vi "Menu-status.vi"(6 "File and Help Menu":bool, 7 "Menu Refnum":refnum<k9>, 8 "Temperature Controller Initialized":bool, 9 "Stage Initialized":bool, 10 "Monochromator Initialized":bool, 11 "CCD Initialized":bool) -> ()   [LabVIEW 2009]
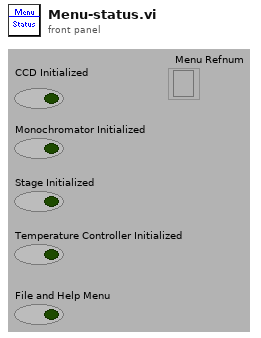
[diagram p1: front panel]
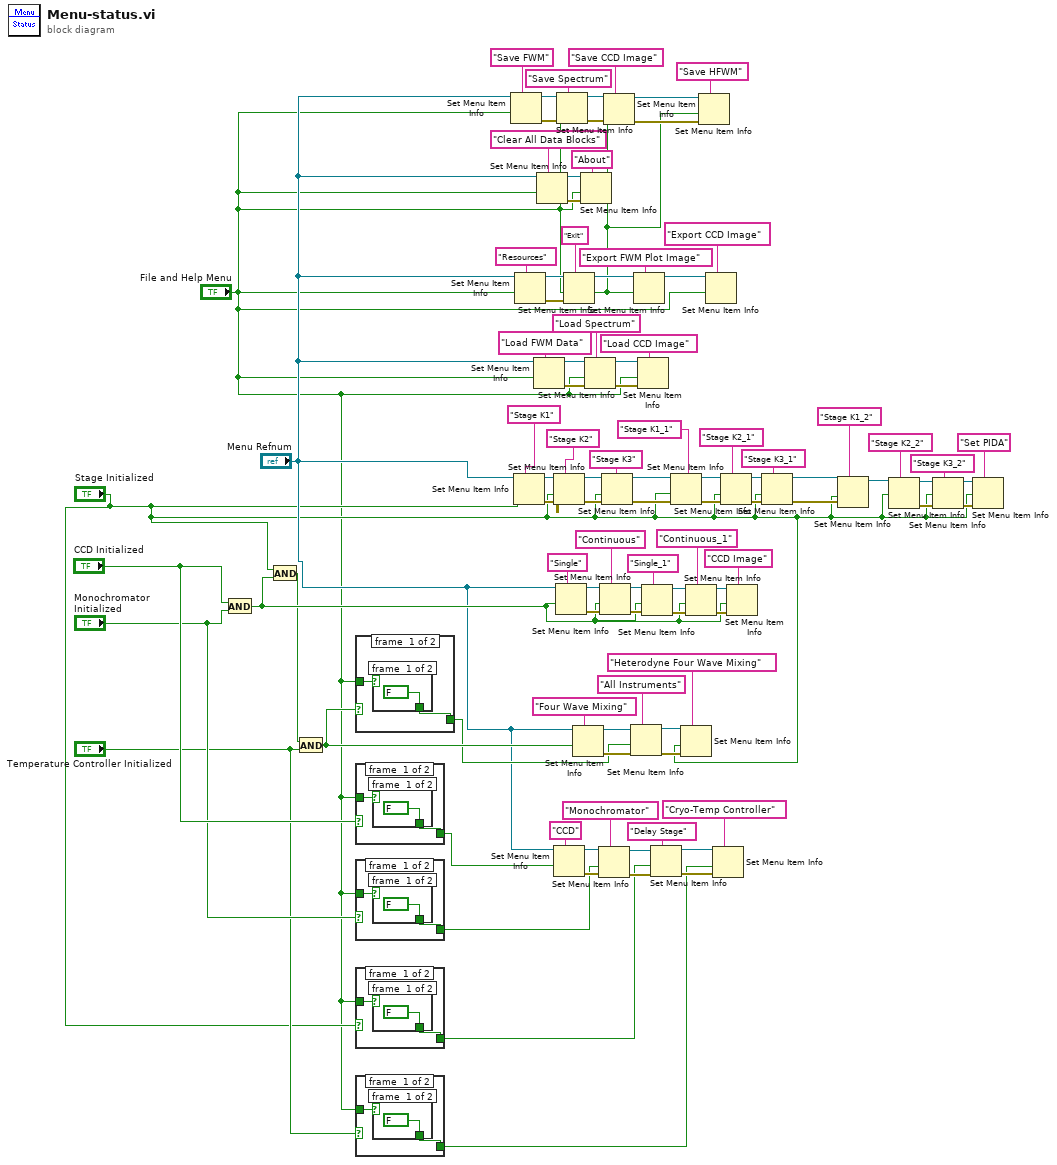
[diagram p0: block diagram]
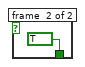
[diagram p2: hidden frame]
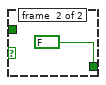
[diagram p3: hidden frame]
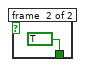
[diagram p4: hidden frame]
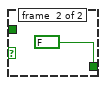
[diagram p5: hidden frame]
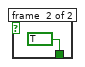
[diagram p6: hidden frame]
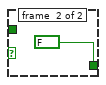
[diagram p7: hidden frame]
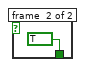
[diagram p8: hidden frame]
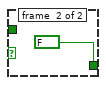
[diagram p9: hidden frame]
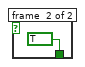
[diagram p10: hidden frame]
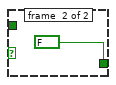
[diagram p11: hidden frame]
diagram:
  n1 = And(x="CCD Initialized", y="Monochromator Initialized") -> (x .and. y?=w64:bool)
  n2 = And(x="Stage Initialized", y=w64) -> (x .and. y?=w63:bool)
  n3 = And(x=w63, y="Temperature Controller Initialized") -> (x .and. y?=w26:bool)
  n4 = case shown="False" w26 {
    tunnel: "File and Help Menu" -> [w101 _]
    tunnel: [w100 FALSE] -> w25
    frame #0 {
      n5 = case shown="True" w101 {
        tunnel: [FALSE TRUE] -> w100
        frame #0 {
        }
        frame #1 {
        }
      }
    }
    frame #1 {
    }
  }
  n6 = case shown="False" "CCD Initialized" {
    tunnel: "File and Help Menu" -> [w106 _]
    tunnel: [w105 FALSE] -> w23
    frame #0 {
      n7 = case shown="True" w106 {
        tunnel: [FALSE TRUE] -> w105
        frame #0 {
        }
        frame #1 {
        }
      }
    }
    frame #1 {
    }
  }
  n8 = case shown="False" "Monochromator Initialized" {
    tunnel: "File and Help Menu" -> [w111 _]
    tunnel: [w110 FALSE] -> w21
    frame #0 {
      n9 = case shown="True" w111 {
        tunnel: [FALSE TRUE] -> w110
        frame #0 {
        }
        frame #1 {
        }
      }
    }
    frame #1 {
    }
  }
  n10 = case shown="False" "Stage Initialized" {
    tunnel: "File and Help Menu" -> [w116 _]
    tunnel: [w115 FALSE] -> w20
    frame #0 {
      n11 = case shown="True" w116 {
        tunnel: [FALSE TRUE] -> w115
        frame #0 {
        }
        frame #1 {
        }
      }
    }
    frame #1 {
    }
  }
  n12 = case shown="False" "Temperature Controller Initialized" {
    tunnel: "File and Help Menu" -> [w121 _]
    tunnel: [w120 FALSE] -> w18
    frame #0 {
      n13 = case shown="True" w121 {
        tunnel: [FALSE TRUE] -> w120
        frame #0 {
        }
        frame #1 {
        }
      }
    }
    frame #1 {
    }
  }
  n14 = Set Menu Item Info(7:"Save FWM" ("item tag"), 9:"File and Help Menu", 11:"Menu Refnum") -> (0:w29:errorcluster, 3:w34:refnum<k9>)  [unwired: 4 in]
  n15 = Set Menu Item Info(7:"Stage K1" ("item tag"), 9:"Stage Initialized", 11:"Menu Refnum") -> (0:w14:errorcluster, 3:w15:refnum<k9>)  [unwired: 4 in]
  n16 = Set Menu Item Info(7:"Resources" ("item tag"), 9:"File and Help Menu", 11:"Menu Refnum") -> (0:w49:errorcluster, 3:w50:refnum<k9>)  [unwired: 4 in]
  n17 = Set Menu Item Info(7:"Load FWM Data" ("item tag"), 9:"File and Help Menu", 11:"Menu Refnum") -> (0:w45:errorcluster, 3:w46:refnum<k9>)  [unwired: 4 in]
  n18 = Set Menu Item Info(7:"Clear All Data Blocks" ("item tag"), 9:"File and Help Menu", 11:"Menu Refnum") -> (0:w27:errorcluster, 3:w30:refnum<k9>)  [unwired: 4 in]
  n19 = Set Menu Item Info(7:"Stage K2" ("item tag"), 8:w14, 9:"Stage Initialized", 11:w15) -> (0:w98:errorcluster, 3:w97:refnum<k9>)  [unwired: 3 in]
  n20 = Set Menu Item Info(7:"CCD" ("item tag"), 9:w23, 11:"Menu Refnum") -> (0:w55:errorcluster, 3:w58:refnum<k9>)  [unwired: 4 in]
  n21 = Set Menu Item Info(7:"Single" ("item tag"), 9:w64, 11:"Menu Refnum") -> (0:w83:errorcluster, 3:w84:refnum<k9>)  [unwired: 4 in]
  n22 = Set Menu Item Info(7:"Save Spectrum" ("item tag"), 8:w29, 9:"File and Help Menu", 11:w34) -> (0:w28:errorcluster, 3:w33:refnum<k9>)  [unwired: 3 in]
  n23 = Set Menu Item Info(7:"Exit" ("item tag"), 8:w49, 9:"File and Help Menu", 11:w50) -> (3:w38:refnum<k9>)  [unwired: 3 in, 1 out]
  n24 = Set Menu Item Info(7:"Four Wave Mixing" ("item tag"), 9:w26, 11:"Menu Refnum") -> (0:w70:errorcluster, 3:w66:refnum<k9>)  [unwired: 4 in]
  n25 = Set Menu Item Info(7:"About" ("item tag"), 8:w27, 9:"File and Help Menu", 11:w30) -> ()  [unwired: 3 in, 2 out]
  n26 = Set Menu Item Info(7:"Load Spectrum" ("item tag"), 8:w45, 9:"File and Help Menu", 11:w46) -> (0:w42:errorcluster, 3:w43:refnum<k9>)  [unwired: 3 in]
  n27 = Set Menu Item Info(7:"Monochromator" ("item tag"), 8:w55, 9:w21, 11:w58) -> (0:w54:errorcluster, 3:w57:refnum<k9>)  [unwired: 3 in]
  n28 = Set Menu Item Info(7:"Continuous" ("item tag"), 8:w83, 9:w64, 11:w84) -> (0:w82:errorcluster, 3:w76:refnum<k9>)  [unwired: 3 in]
  n29 = Set Menu Item Info(7:"Stage K3" ("item tag"), 8:w98, 9:"Stage Initialized", 11:w97) -> (0:w13:errorcluster, 3:w11:refnum<k9>)  [unwired: 3 in]
  n30 = Set Menu Item Info(7:"Save CCD Image" ("item tag"), 8:w28, 9:"File and Help Menu", 11:w33) -> (0:w3:errorcluster, 3:w2:refnum<k9>)  [unwired: 3 in]
  n31 = Set Menu Item Info(7:"All Instruments", 9:w25, 11:w66) -> (3:w65:refnum<k9>)  [unwired: 4 in, 1 out]
  n32 = Set Menu Item Info(7:"Export FWM Plot Image" ("item tag"), 9:"File and Help Menu", 11:w38) -> (3:w39:refnum<k9>)  [unwired: 4 in, 1 out]
  n33 = Set Menu Item Info(7:"Load CCD Image" ("item tag"), 8:w42, 9:"File and Help Menu", 11:w43) -> ()  [unwired: 3 in, 2 out]
  n34 = Set Menu Item Info(7:"Single_1" ("item tag"), 8:w82, 9:w64, 11:w76) -> (0:w81:errorcluster, 3:w75:refnum<k9>)  [unwired: 3 in]
  n35 = Set Menu Item Info(7:"Delay Stage" ("item tag"), 8:w54, 9:w20, 11:w57) -> (0:w53:errorcluster, 3:w56:refnum<k9>)  [unwired: 3 in]
  n36 = Set Menu Item Info(7:"Stage K1_1" ("item tag"), 8:w13, 9:"Stage Initialized", 11:w11) -> (0:w12:errorcluster, 3:w10:refnum<k9>)  [unwired: 3 in]
  n37 = Set Menu Item Info(7:"Heterodyne Four Wave Mixing" ("item tag"), 8:w70, 9:"Stage Initialized", 11:w65) -> ()  [unwired: 3 in, 2 out]
  n38 = Set Menu Item Info(7:"Continuous_1" ("item tag"), 8:w81, 9:w64, 11:w75) -> (0:w74:errorcluster, 3:w73:refnum<k9>)  [unwired: 3 in]
  n39 = Set Menu Item Info(7:"Save HFWM" ("item tag"), 8:w3, 9:"File and Help Menu", 11:w2) -> ()  [unwired: 3 in, 2 out]
  n40 = Set Menu Item Info(7:"Export CCD Image" ("item tag"), 9:"File and Help Menu", 11:w39) -> ()  [unwired: 4 in, 2 out]
  n41 = Set Menu Item Info(7:"Cryo-Temp Controller", 8:w53, 9:w18, 11:w56) -> ()  [unwired: 3 in, 2 out]
  n42 = Set Menu Item Info(7:"Stage K2_1" ("item tag"), 8:w12, 9:"Stage Initialized", 11:w10) -> (0:w94:errorcluster, 3:w93:refnum<k9>)  [unwired: 3 in]
  n43 = Set Menu Item Info(7:"CCD Image" ("item tag"), 8:w74, 9:w64, 11:w73) -> ()  [unwired: 3 in, 2 out]
  n44 = Set Menu Item Info(7:"Stage K3_1" ("item tag"), 8:w94, 9:"Stage Initialized", 11:w93) -> (0:w8:errorcluster, 3:w7:refnum<k9>)  [unwired: 3 in]
  n45 = Set Menu Item Info(7:"Stage K1_2" ("item tag"), 8:w8, 9:"Stage Initialized", 11:w7) -> (3:w6:refnum<k9>)  [unwired: 3 in, 1 out]
  n46 = Set Menu Item Info(7:"Stage K2_2" ("item tag"), 9:"Stage Initialized", 11:w6) -> (0:w90:errorcluster, 3:w89:refnum<k9>)  [unwired: 4 in]
  n47 = Set Menu Item Info(7:"Stage K3_2" ("item tag"), 8:w90, 9:"Stage Initialized", 11:w89) -> (0:w87:errorcluster, 3:w86:refnum<k9>)  [unwired: 3 in]
  n48 = Set Menu Item Info(7:"Set PIDA" ("item tag"), 8:w87, 9:"Stage Initialized", 11:w86) -> ()  [unwired: 3 in, 2 out]
